vi "InitTabFocus.vi"(8 "error in (no error)":errorcluster, 11 "GuiderSetup in":refnum<class "GuiderSetup.lvclass">) -> (0 "error out":errorcluster, 2 "output cluster":T1, 3 "GuiderSetup out":refnum<class "GuiderSetup.lvclass">)   [LabVIEW 2018, in "GuiderSetup.lvclass"]
uses:
  GuiderSetup.lvclass
  C:/Users/devstaff/sparc4/s4gui/Versao ZeroMQ REQ-REP/SPARC4_GUI -v1.0.0 - 20241216/S4GUI/S4GUI.lvclass
  S4GUI/S4GUI.lvclass/S4GUI.ctl
  <vilib>/Utility/config.llb/Read Key (Double).vi
  Instrument/Instrument.lvclass
  S4GUI/S4GUI.lvclass
  <vilib>/Utility/config.llb/NI_LVConfig.lvlib
panel:
  in  "Focus by Mode":T1={"Phot."=17.0, "Polarim"=7.0, "Efficiency"=0.0, "Instrumental"=0.0}
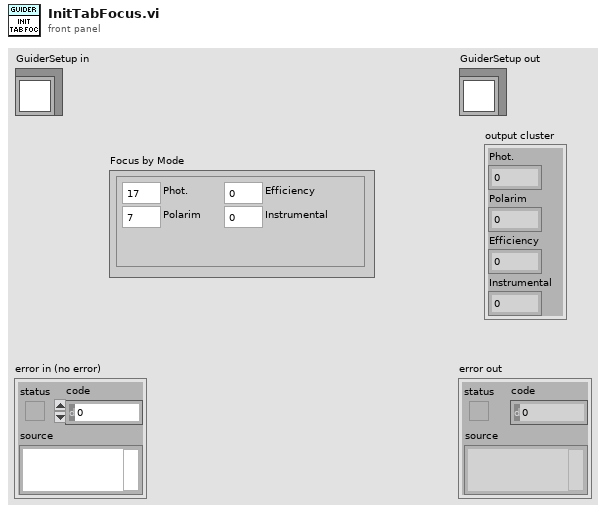
[diagram p1: front panel]
types:
  T1 = cluster{"Phot.":dbl, "Polarim":dbl, "Efficiency":dbl, "Instrumental":dbl}
  T2 = typedef "NI_LVConfig.lvlib/Config Data RefNum.ctl" = refnum<k1>
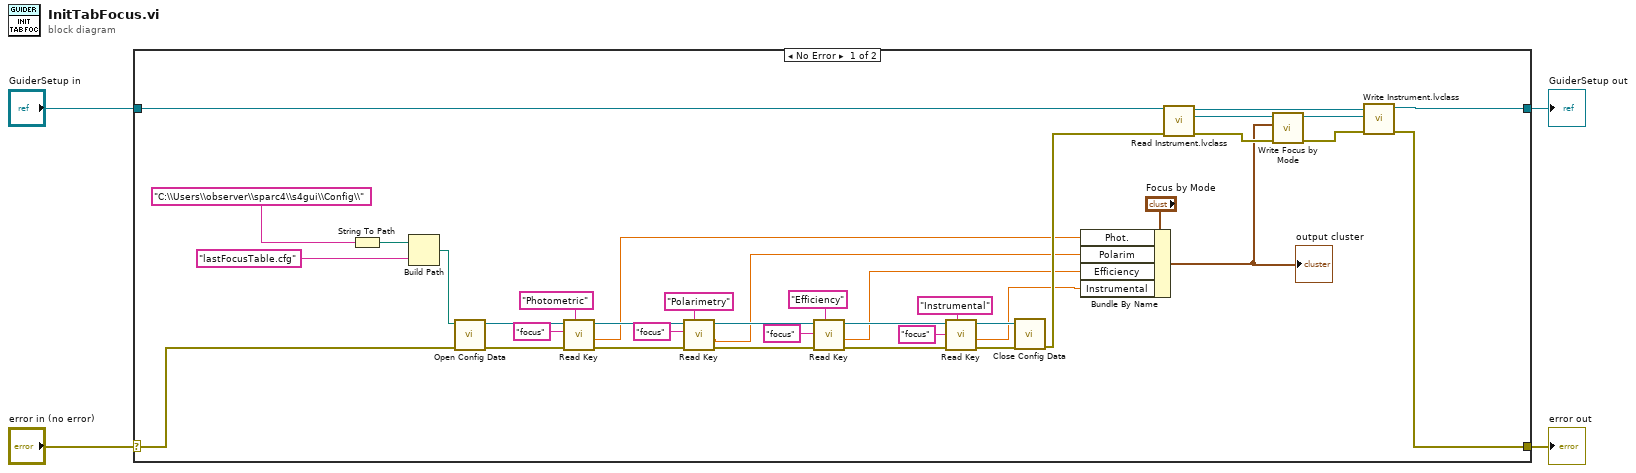
[diagram p0: block diagram]
diagram:
  n1 = case shown="No Error" "error in (no error)" {
    selector: "error in (no error)" -> [w11 w44]
    tunnel: [w35 w44] -> w3
    tunnel: [w38 w43] -> w1
    tunnel: "GuiderSetup in" -> [w39 w43]
    frame No Error {
      n2 = String To Path(string="C:\\Users\\observer\\sparc4\\s4gui\\Config\\") -> (path=w24:path)
      n3 = Build Path(base path=w24, name or relative path="lastFocusTable.cfg") -> (appended path=w21:path)
      n4 = call <vilib>:"Open Config Data.vi"("error in (no error)"=w11, "configuration file path"=w21) -> ("error out"=w23:errorcluster, "refnum"=w22:T2)  [unwired: 7 in, 1 out]
      n5 = call-poly <vilib>:"Read Key.vi"("section"="Photometric" ("key"), "error in (no error)"=w23, "key"="focus", "refnum"=w22) -> ("error out"=w27:errorcluster, "value"=w8:dbl, "refnum out"=w25:T2)  [unwired: 4 in, 1 out]
      n6 = call-poly <vilib>:"Read Key.vi"("section"="Polarimetry" ("key"), "error in (no error)"=w27, "key"="focus", "refnum"=w25) -> ("error out"=w28:errorcluster, "value"=w7:dbl, "refnum out"=w26:T2)  [unwired: 4 in, 1 out]
      n7 = call-poly <vilib>:"Read Key.vi"("section"="Efficiency" ("key"), "error in (no error)"=w28, "key"="focus", "refnum"=w26) -> ("error out"=w31:errorcluster, "value"=w6:dbl, "refnum out"=w29:T2)  [unwired: 4 in, 1 out]
      n8 = call-poly <vilib>:"Read Key.vi"("section"="Instrumental" ("key"), "error in (no error)"=w31, "key"="focus", "refnum"=w29) -> ("error out"=w32:errorcluster, "value"=w9:dbl, "refnum out"=w30:T2)  [unwired: 4 in, 1 out]
      n9 = call <vilib>:"Close Config Data.vi"("error in (no error)"=w32, "refnum"=w30) -> ("error out"=w10:errorcluster)  [unwired: 8 in, 1 out]
      n10 = Bundle By Name(cluster="Focus by Mode", "Phot."=w8, "Polarim"=w7, "Efficiency"=w6, "Instrumental"=w9) -> (w33:T1)
      "output cluster" <- w33
      n11 = call "Read Instrument.lvclass.vi"("error in (no error)"=w10, "S4ACS_GUI in"=w39) -> ("error out"=w37:errorcluster, "Instrument.lvclass"=w41:refnum<class "Instrument.lvclass">, "S4ACS_GUI out"=w42:refnum<class "GuiderSetup.lvclass">)  [unwired: 7 in]
      n12 = call-dynamic "Write Focus by Mode.vi"("error in (no error)"=w37, "Focus by Mode"=w33, "Instrument in"=w41) -> ("error out"=w36:errorcluster, "Instrument out"=w40:refnum<class "Instrument.lvclass">)  [unwired: 7 in]
      n13 = call "Write Instrument.lvclass.vi"("error in (no error)"=w36, "Instrument.lvclass"=w40, "S4ACS_GUI in"=w42) -> ("error out"=w35:errorcluster, "S4ACS_GUI out"=w38:refnum<class "GuiderSetup.lvclass">)  [unwired: 7 in]
    }
    frame Error {
    }
  }
  "error out" <- w3
  "GuiderSetup out" <- w1
